vi "Input_raw.vi"(0 "Current * 10^input":dbl, 3 "Sensitivity":dbl, 5 "Drag":dbl, 7 "Signal in":dbl, 11 "Frame Properties (Remapped)":T1) -> (1 "Scaled Current":dbl, 2 "feedback":bool)   [LabVIEW 2019]
uses:
  <userlib>/HapticSTM/HapticSTM.lvlib
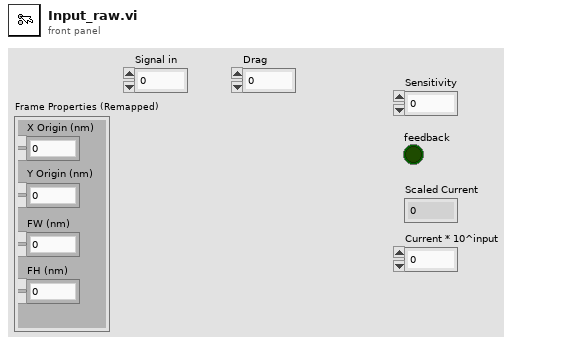
[diagram p1: front panel]
types:
  T1 = cluster{"X Origin (nm)":dbl, "Y Origin (nm)":dbl, "FW (nm)":dbl, "FH (nm)":dbl}
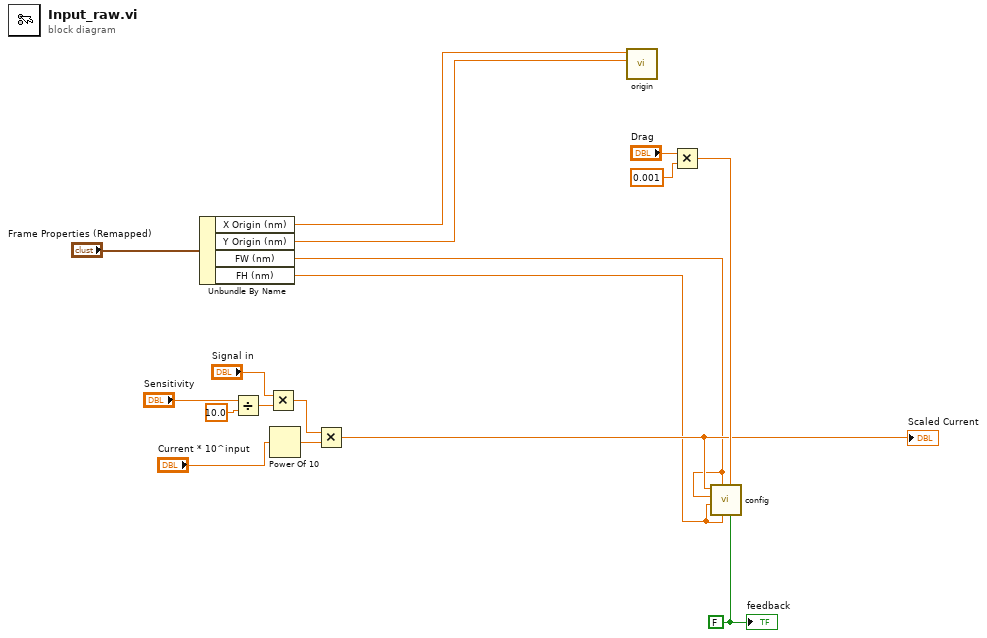
[diagram p0: block diagram]
diagram:
  w11 = FALSE ("feedback")
  n1 = Unbundle By Name("Frame Properties (Remapped)") -> ("X Origin (nm)"=w4:dbl, "Y Origin (nm)"=w3:dbl, "FW (nm)"=w2:dbl, "FH (nm)"=w1:dbl)
  n2 = Divide(x="Sensitivity", y=10.0) -> (x/y=w8:dbl)
  n3 = Multiply(x="Signal in", y=w8) -> (x*y=w9:dbl)
  n4 = Power Of 10(x="Current * 10^input") -> (10^x=w13:dbl)
  n5 = Multiply(x=w9, y=w13) -> (x*y=w12:dbl)
  "Scaled Current" <- w12
  n6 = call <userlib>:"origin.vi"("zorg"=w3, "xorg"=w4) -> ()  [unwired: 10 in]
  n7 = Multiply(x="Drag", y=0.001) -> (x*y=w15:dbl)
  n8 = call <userlib>:"config.vi"("feedback"=w11, "dragc"=w15, "sizeofimgz"=w1, "sizeofimgx"=w2, "scopez"=w1, "scopex"=w2, "ypos"=w12) -> ()  [unwired: 5 in]
  "feedback" <- w11
